vi "Get Create Temporary Images.vi"(8 "error in (no error)":errorcluster, 10 "Image in":T1, 11 "Analyze BaseClass in":refnum<class "Analyze BaseClass.lvclass">) -> (0 "error out":errorcluster, 1 "image mask":T1, 2 "work image":T1, 3 "Analyze BaseClass out":refnum<class "Analyze BaseClass.lvclass">, 5 "masked image":T1)   [LabVIEW 2014, in "Analyze.lvlib" / "Analyze BaseClass.lvlib" / "Analyze BaseClass.lvclass"]
uses:
  Analyze BaseClass.lvclass
  <vilib>/vision/Image Controls.llb/IMAQ Image.ctl
  Analyze BaseClass.lvclass/Analyze BaseClass.ctl
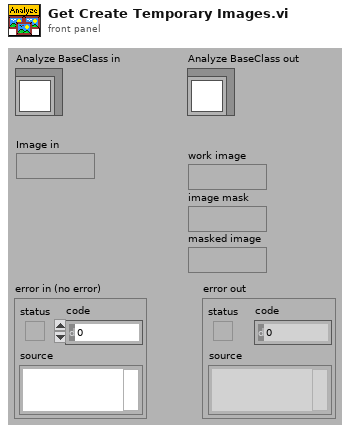
[diagram p1: front panel]
types:
  T1 = typedef "IMAQ Image.ctl" = refnum<image>
  T2 = typedef "Image Type" = u32
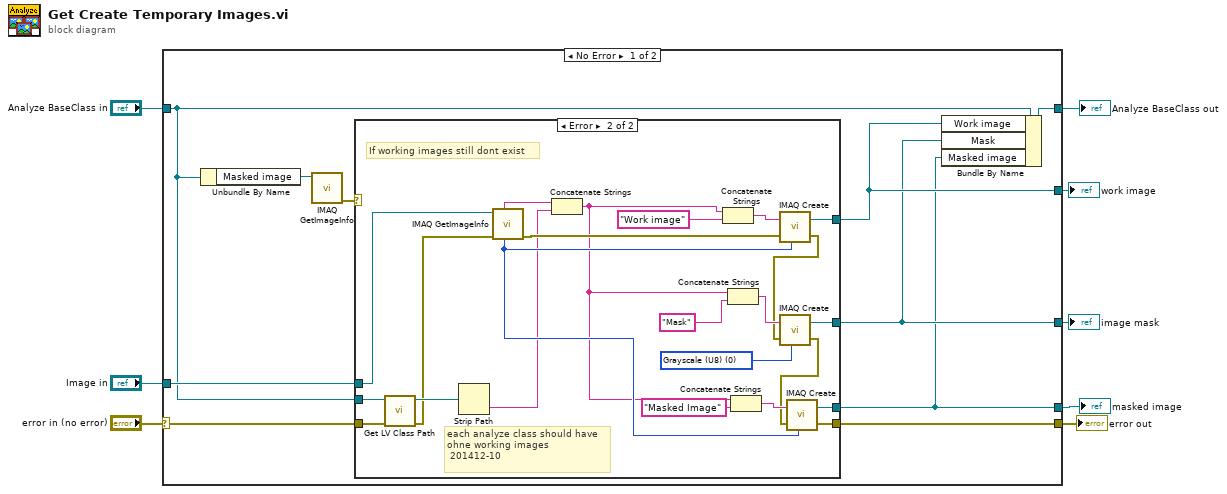
[diagram p0: block diagram]
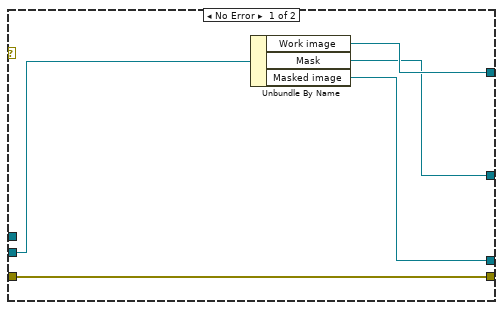
[diagram p2: hidden frame]
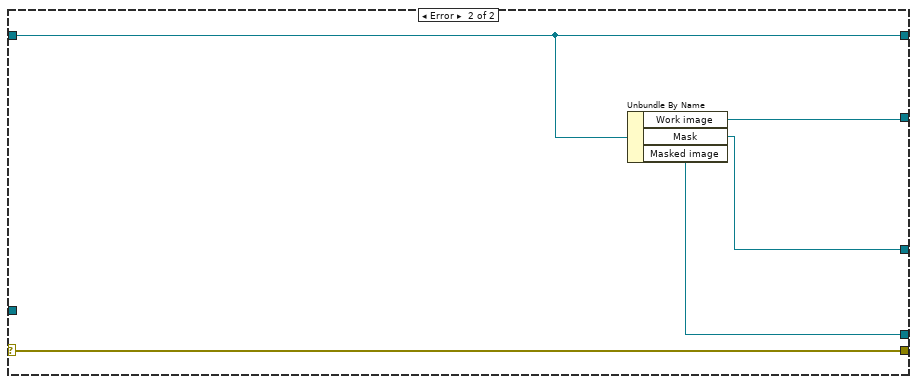
[diagram p3: hidden frame]
diagram:
  n1 = case shown="No Error" "error in (no error)" {
    selector: "error in (no error)" -> [w9 w51]
    tunnel: [w15 w51] -> w7
    tunnel: [w14 w50] -> w5
    tunnel: "Analyze BaseClass in" -> [w10 w50]
    tunnel: "Image in" -> [w16 _]
    tunnel: [w13 w49] -> w3
    tunnel: [w12 w48] -> w2
    tunnel: [w11 w47] -> w1
    frame No Error {
      n2 = Unbundle By Name(w10) -> ("Masked image"=w17:T1)
      n3 = call "IMAQ GetImageInfo"("Image"=w17) -> ("error out"=w18:errorcluster)  [unwired: 3 in, 7 out]
      n4 = case shown="Error" w18 {
        tunnel: [w22 w46] -> w13
        tunnel: [w20 w42] -> w11
        tunnel: [w21 w41] -> w12
        tunnel: w16 -> [_ w24]
        tunnel: [w19 w31] -> w15
        tunnel: w10 -> [w23 w28]
        tunnel: w9 -> [w19 w29]
        frame No Error {
          n5 = Unbundle By Name(w23) -> ("Work image"=w22:T1, "Mask"=w21:T1, "Masked image"=w20:T1)
        }
        frame Error {
          w44 = T2 0 items=["Grayscale (U8)", "Grayscale (I16)", "Grayscale (SGL)", "Complex (CSG)", "RGB (U32)", "HSL (U32)", "RGB (U64)", "Grayscale (U16)"] ("Image Type")
          # "each analyze class should have\nohne working images\n 201412-10"
          # "If working images still dont exist"
          n6 = call <vilib>:"Get LV Class Path.vi"("error in (no error)"=w29, "object"=w28) -> ("error out"=w27:errorcluster, "class path"=w30:path)  [unwired: 8 in]
          n7 = Strip Path(path=w30) -> (name=w25:string)  [unwired: 1 out]
          n8 = call "IMAQ GetImageInfo"("error in (no error)"=w27, "Image"=w24) -> ("error out"=w34:errorcluster, "Image Name"=w36:string, "Image Type"=w35:T2)  [unwired: 2 in, 5 out]
          n9 = Concatenate Strings(w36, w25) -> (w26:string)
          n10 = Concatenate Strings(w26, "Work image" ("Image Name")) -> (w40:string)
          n11 = Concatenate Strings(w26, "Mask" ("Image Name")) -> (w38:string)
          n12 = Concatenate Strings(w26, "Masked Image" ("Image Name")) -> (w37:string)
          n13 = call "IMAQ Create"("Image Name"=w40, "Image Type"=w35, "error in (no error)"=w34) -> ("New Image"=w46:T1, "error out"=w33:errorcluster)  [unwired: 2 in]
          n14 = call "IMAQ Create"("Image Name"=w38, "Image Type"=w44, "error in (no error)"=w33) -> ("New Image"=w41:T1, "error out"=w32:errorcluster)  [unwired: 2 in]
          n15 = call "IMAQ Create"("Image Name"=w37, "Image Type"=w35, "error in (no error)"=w32) -> ("New Image"=w42:T1, "error out"=w31:errorcluster)  [unwired: 2 in]
        }
      }
      n16 = Bundle By Name(cluster=w10, "Work image"=w13, "Mask"=w12, "Masked image"=w11) -> (w14:refnum<class "Analyze BaseClass.lvclass">)
    }
    frame Error {
      n17 = Unbundle By Name(w50) -> ("Work image"=w49:T1, "Mask"=w48:T1, "Masked image"=w47:T1)
    }
  }
  "error out" <- w7
  "Analyze BaseClass out" <- w5
  "work image" <- w3
  "image mask" <- w2
  "masked image" <- w1
